vi "Details.vi"() -> ()   [LabVIEW 2020]
uses:
  Controls/Basic Pump Params.ctl
  Controls/Pump Phases.ctl
  Controls/SImulation Data.ctl
  SubVIs/Pump Global Variables.vi
panel:
  in  "Boolean":bool
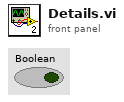
[diagram p1: front panel]
types:
  T1 = typedef "SImulation Data.ctl" = cluster{"Time Stamp":timestamp, "Solution":string, "Volume Dispensed":string}
  T2 = typedef "Pump Phases.ctl" = cluster{"Valve Position":sgl, "Solution Name":string, "Pump Rate":dbl, "Target Time":dbl, "Target Volume":dbl}
  T3 = typedef "Basic Pump Params.ctl" = cluster{"Diameter (mm)":dbl, "Pump Direction":string, "Target Time 12":dbl, "Units 2":string}
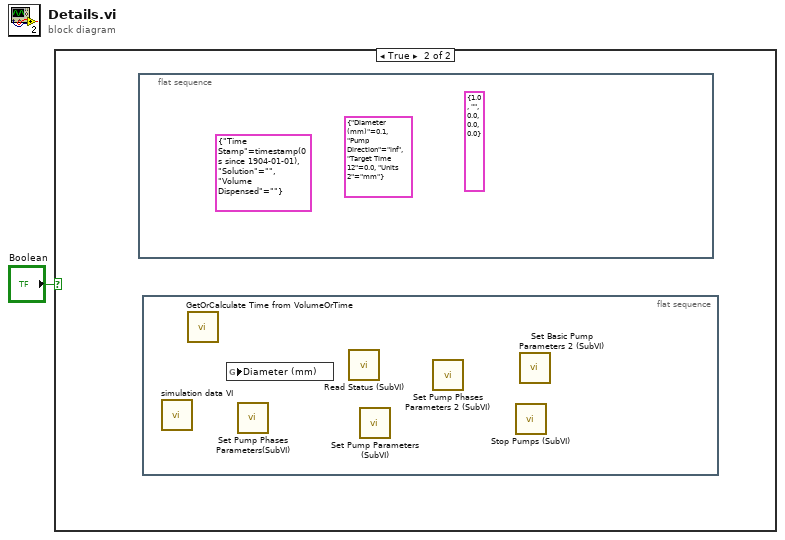
[diagram p0: block diagram]
diagram:
  n1 = case shown="True" "Boolean" {
    frame False {
    }
    frame True {
      n2 = flat-sequence {
        frame #0 {
          (unwired) T1 {"Time Stamp"=timestamp(0 s since 1904-01-01), "Solution"="", "Volume Dispensed"=""} ("Cluster")
          (unwired) T2 {"Valve Position"=1.0, "Solution Name"="", "Pump Rate"=0.0, "Target Time"=0.0, "Target Volume"=0.0} ("Cluster")
          (unwired) T3 {"Diameter (mm)"=0.1, "Pump Direction"="inf", "Target Time 12"=0.0, "Units 2"="mm"} ("Basic Data")
        }
      }
      n3 = flat-sequence {
        frame #0 {
          n4 = call "simulation data VI.vi"() -> ()  [unwired: 4 in, 1 out]
          n5 = call "GetOrCalculate Time from VolumeOrTime.vi"() -> ()  [unwired: 5 in, 1 out]
          n6 = global read "Pump Global Variables.vi" "Diameter (mm)"() -> ()  [unwired: 1 in]
          n7 = call "Set Pump Phases Parameters(SubVI).vi"() -> ()  [unwired: 7 in, 2 out]
          n8 = call "Read Status (SubVI).vi"() -> ()  [unwired: 4 in, 3 out]
          n9 = call "Set Pump Parameters (SubVI).vi"() -> ()  [unwired: 9 in, 2 out]
          n10 = call "Set Pump Phases Parameters 2 (SubVI).vi"() -> ()  [unwired: 10 in, 2 out]
          n11 = call "Stop Pumps (SubVI).vi"() -> ()  [unwired: 2 in, 2 out]
          n12 = call "Set Basic Pump Parameters 2 (SubVI).vi"() -> ()  [unwired: 9 in, 2 out]
        }
      }
    }
  }
